vi "Execute.vi"(0 "object in":refnum<class "Viewer.lvclass">, 2 "Requirements":T2={"From"=enum."TDMS", "File Handler"=variant, "Input"=variant(map{string, dbl[]} {})}, 5 "Error In":errorcluster) -> (14 "object out":refnum<class "Viewer.lvclass">, 16 "Message":T1, 19 "Error Out":errorcluster)   [LabVIEW 2024, in "Viewer.lvclass"]
doc: "Opens the file and returns data inside with Message type definition's data variant"
uses:
  Viewer.lvclass
  Support/Type Def/Requirements.ctl
  Support/Type Def/Message.ctl
  Support/Type Def/Data.ctl
  <vilib>/Utility/file.llb/Read Delimited Spreadsheet (DBL).vi
  Viewer.lvclass/Viewer.ctl
panel:
  # "Connector Pane"
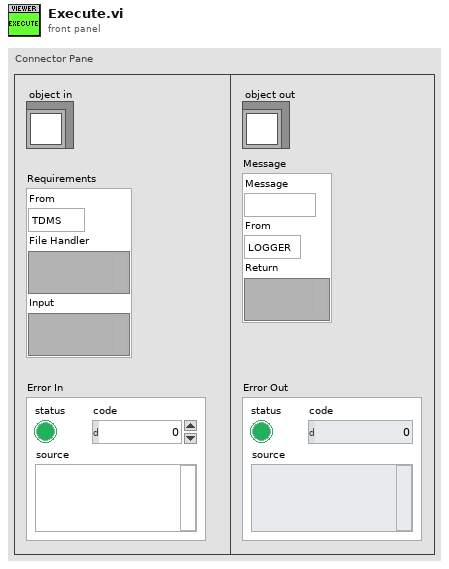
[diagram p1: front panel]
types:
  T1 = typedef "Message.ctl" = cluster{"Message":string, "From":enum16{"LOGGER", "VIEWER"}, "Return":variant}
  T2 = typedef "Requirements.ctl" = cluster{"From":enum16{"TDMS", "EXCEL"}, "File Handler":variant, "Input":variant}
  T3 = typedef "Data.ctl" = map{string, dbl[]}
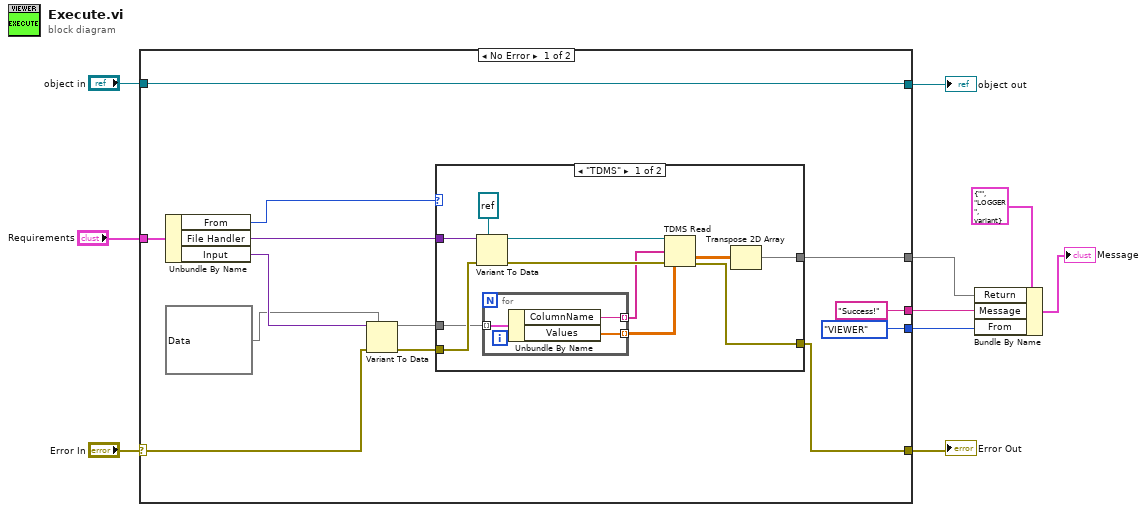
[diagram p0: block diagram]
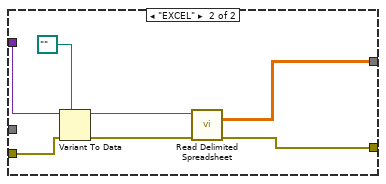
[diagram p2: hidden frame]
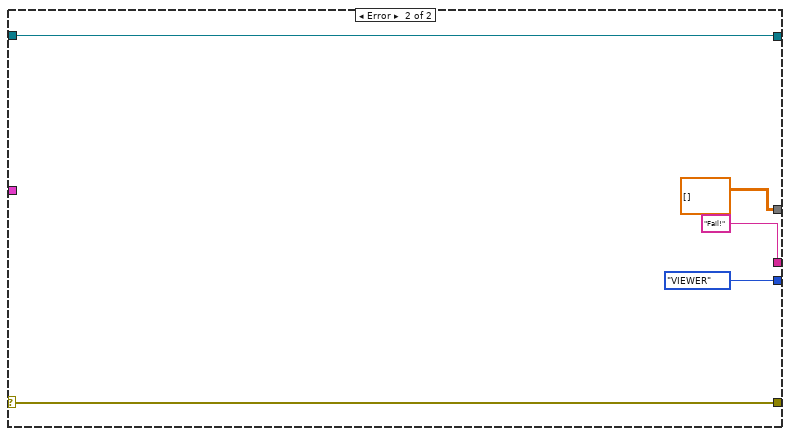
[diagram p3: hidden frame]
diagram:
  n1 = case shown="No Error" "Error In" {
    selector: "Error In" -> [w15 w49]
    tunnel: [w11 w49] -> w9
    tunnel: [w23 w48] -> w7
    tunnel: "object in" -> [w23 w48]
    tunnel: "Requirements" -> [w22 _]
    tunnel: [w19 dbl[][] [] ("all rows")] -> w3
    tunnel: ["Success!" ("Message") "Fail!" ("Message")] -> w2
    tunnel: [enum16{"LOGGER", "VIEWER"}."VIEWER" ("From") enum16{"LOGGER", "VIEWER"}."VIEWER" ("From")] -> w1
    frame No Error {
      n2 = Unbundle By Name(w22) -> ("From"=w21:enum16{"TDMS", "EXCEL"}, "File Handler"=w20:variant, "Input"=w16:variant)
      n3 = Variant To Data(error in=w15, type=T3 {} ("Data"), Variant=w16) -> (data=w13:T3, error out=w14:errorcluster)
      n4 = case shown="\"TDMS\"" w21 {
        tunnel: w20 -> [w33 w42]
        tunnel: [w24 w40] -> w19
        tunnel: w14 -> [w30 w38]
        tunnel: w13 -> [w29 _]
        tunnel: [w27 w39] -> w11
        frame "TDMS" {
          n5 = Variant To Data(error in=w30, type=refnum<k34> refnum ("tdms file"), Variant=w33) -> (data=w31:refnum<k34>, error out=w32:errorcluster)
          n6 = for {
            tunnel: w29 -> [w37] mode=indexing
            tunnel: [w36] -> w26 mode=indexing
            tunnel: [w35] -> w25 mode=indexing
            n7 = Unbundle By Name(w37) -> ("ColumnName"=w35:string, "Values"=w36:dbl[])
          }
          n8 = TDMS Read(0:w31, 7:w25, 11:w32, 12:w26) -> (10:w28:dbl[][], 15:w27:errorcluster)  [unwired: 4 in, 4 out]
          n9 = Transpose 2D Array(2D array=w28) -> (transposed array=w24:dbl[][])
        }
        frame "EXCEL" {
          n10 = Variant To Data(error in=w38, type=path "" ("file path (dialog if empty)"), Variant=w42) -> (data=w41:path, error out=w44:errorcluster)
          n11 = call-poly <vilib>:"Read Delimited Spreadsheet.vi"("file path (dialog if empty)"=w41, "error in (no error)"=w44) -> ("all rows"=w40:dbl[][], "error out"=w39:errorcluster)  [unwired: 8 in, 4 out]
        }
      }
    }
    frame Error {
    }
  }
  "Error Out" <- w9
  "object out" <- w7
  n12 = Bundle By Name(cluster=T1 {"Message"="", "From"=enum."LOGGER", "Return"=variant} ("Message"), "Return"=w3, "Message"=w2, "From"=w1) -> (→"Message":T1)
